vi "Create GPIO DAQ Task.vi"(8 "error in":errorcluster, 11 "GPIO Channels":T1={"Pin3"="PXI1Slot3/port0/line0", "Pin6"="PXI1Slot3/port0/line3", "Pin7"="PXI1Slot3/port0/line4", "Pin9"="PXI1Slot3/port0/line28", "Pin10"="PXI1Slot3/port0/line10", "Pin11"="PXI1Slot3/port0/line4", "Pin12"="PXI1Slot3/port0/line12", "Pin13"="PXI1Slot3/port0/line15", "Pin14"="PXI1Slot3/port0/line22", "Pin15"="PXI1Slot3/port0/line23", "Pin17"="PXI1Slot3/port0/line26", "Pin18"="PXI1Slot3/port0/line30", "Pin20"="PXI1Slot3/port0/line29", "Pin25"="PXI1Slot3/port0/line19", "Pin26"="PXI1Slot3/port0/line17", "Pin28"="PXI1Slot3/port0/line25", "Pin29"="PXI1Slot3/port1/line3", "Pin30"="PXI1Slot3/port0/line24", "Pin31"="PXI1Slot3/port1/line4"}) -> (0 "error out":errorcluster, 3 "GPIO Task":refnum<k21>)   [LabVIEW 2018]
uses:
  <vilib>/DAQmx/create/channels.llb/DAQmx Create Channel (DI-Digital Input).vi
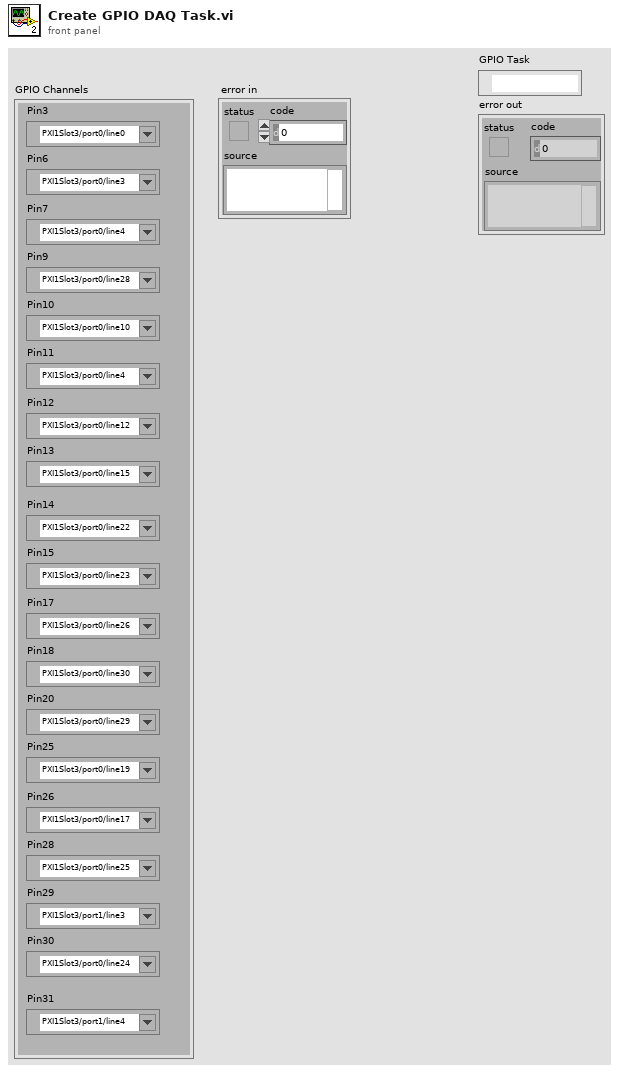
[diagram p1: front panel]
types:
  T1 = cluster{"Pin3":tag, "Pin6":tag, "Pin7":tag, "Pin9":tag, "Pin10":tag, "Pin11":tag, "Pin12":tag, "Pin13":tag, "Pin14":tag, "Pin15":tag, "Pin17":tag, "Pin18":tag, "Pin20":tag, "Pin25":tag, "Pin26":tag, "Pin28":tag, "Pin29":tag, "Pin30":tag, "Pin31":tag}
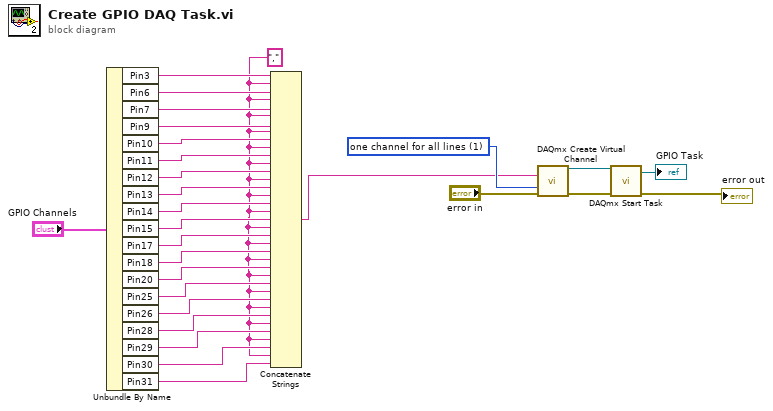
[diagram p0: block diagram]
diagram:
  w3 = "," ("string")
  w28 = 1 items=["one channel for each line", "one channel for all lines"] ("line grouping")
  n1 = Unbundle By Name("GPIO Channels") -> ("Pin3"=w21:tag, "Pin6"=w20:tag, "Pin7"=w19:tag, "Pin9"=w18:tag, "Pin10"=w17:tag, "Pin11"=w16:tag, "Pin12"=w15:tag, "Pin13"=w14:tag, "Pin14"=w13:tag, "Pin15"=w12:tag, "Pin17"=w11:tag, "Pin18"=w10:tag, "Pin20"=w9:tag, "Pin25"=w8:tag, "Pin26"=w7:tag, "Pin28"=w6:tag, "Pin29"=w5:tag, "Pin30"=w4:tag, "Pin31"=w2:tag)
  n2 = Concatenate Strings(w21, w3, w20, w3, w19, w3, w18, w3, w17, w3, w16, w3, w15, w3, w14, w3, w13, w3, w12, w3, w11, w3, w10, w3, w9, w3, w8, w3, w7, w3, w6, w3, w5, w3, w4, w3, w2) -> (w1:string)
  n3 = call-poly <vilib>:"DAQmx Create Virtual Channel.vi"("lines"=w1, "line grouping"=w28, "error in"="error in") -> ("task out"=w26:refnum<k21>, "error out"=w25:errorcluster)  [unwired: 11 in]
  n4 = call <vilib>:"DAQmx Start Task.vi"("task/channels in"=w26, "error in"=w25) -> ("task out"=→"GPIO Task":refnum<k21>, "error out"=→"error out":errorcluster)  [unwired: 12 in]
